vi "_FPGA_StepwiseIncreasing.vi"(7 "Step interval":u32=5000, 9 "Enable ouput":bool, 11 "Target AO":fxp<+,14,14>) -> (1 "Action done?":bool, 3 "AO":fxp<+,14,14>)   [LabVIEW 2018]
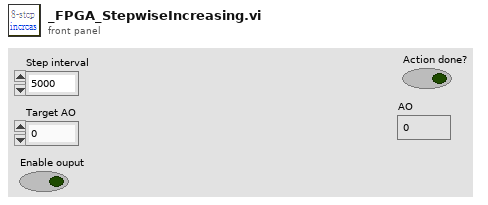
[diagram p1: front panel]
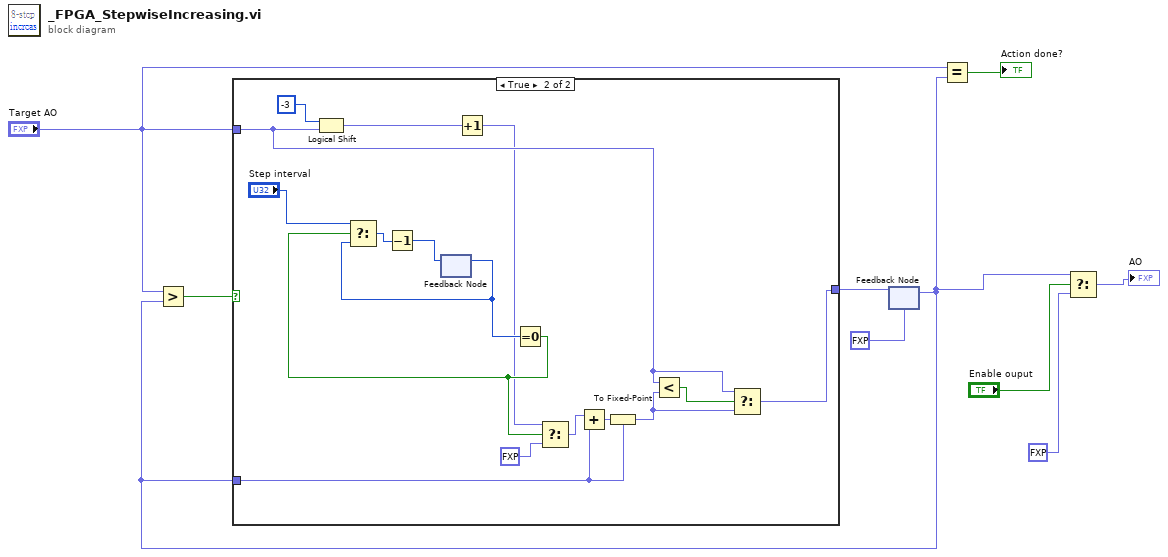
[diagram p0: block diagram]
diagram:
  n1 = feedback #1(fxp<+,14,14> 0.0 ("Target AO")) -> (w3:fxp<+,16,16>)
  n2 = Greater?(x="Target AO", y=w3) -> (0:w9:bool)
  n3 = case shown="True" w9 {
    tunnel: "Target AO" -> [w10 w17]
    tunnel: [w10 w13] -> w2
    tunnel: w3 -> [_ w11]
    frame False {
    }
    frame True {
      n4 = Logical Shift(y=i16 -3, x=w17) -> (x << y=w14:fxp<+,14,14>)
      n5 = feedback #2() -> (w22:u32)  [unwired: 1 in]
      n6 = Increment(x=w14) -> (x+1=w12:fxp<+,15,15>)
      n7 = Equal To 0?(x=w22) -> (x = 0?=w20:bool)
      n8 = Select(t="Step interval", s=w20, f=w22) -> (s? t:f=w24:u32)
      n9 = Decrement(x=w24) -> (x-1=w23:u32)
      n10 = feedback-in #2(w23) -> ()
      n11 = Select(t=w12, s=w20, f=fxp<+,14,14> 0.0) -> (s? t:f=w18:fxp<+,15,15>)
      n12 = Add(x=w18, y=w11) -> (x+y=w16:fxp<+,16,16>)
      n13 = To Fixed-Point(fixed-point type=w11, number=w16) -> (fixed-point=w15:fxp<+,16,16>)
      n14 = Less?(x=w17, y=w15) -> (x < y?=w21:bool)
      n15 = Select(t=w17, s=w21, f=w15) -> (s? t:f=w13:fxp<+,16,16>)
    }
  }
  n16 = feedback-in #1(w2) -> ()
  n17 = Equal?(x="Target AO", y=w3) -> (x = y?=→"Action done?":bool)
  n18 = Select(t=w3, s="Enable ouput", f=fxp<+,14,14> 0.0) -> (s? t:f=→"AO":fxp<+,16,16>)
